vi "Parse Custom Mode (Pixhawk).vi"(8 "Error In":errorcluster, 11 "custom mode":u32) -> (0 "Error Out":errorcluster, 3 "Custom Mode":string)   [LabVIEW 2014]
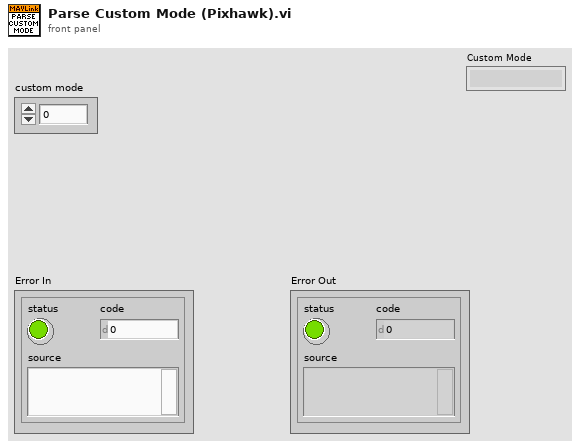
[diagram p1: front panel]
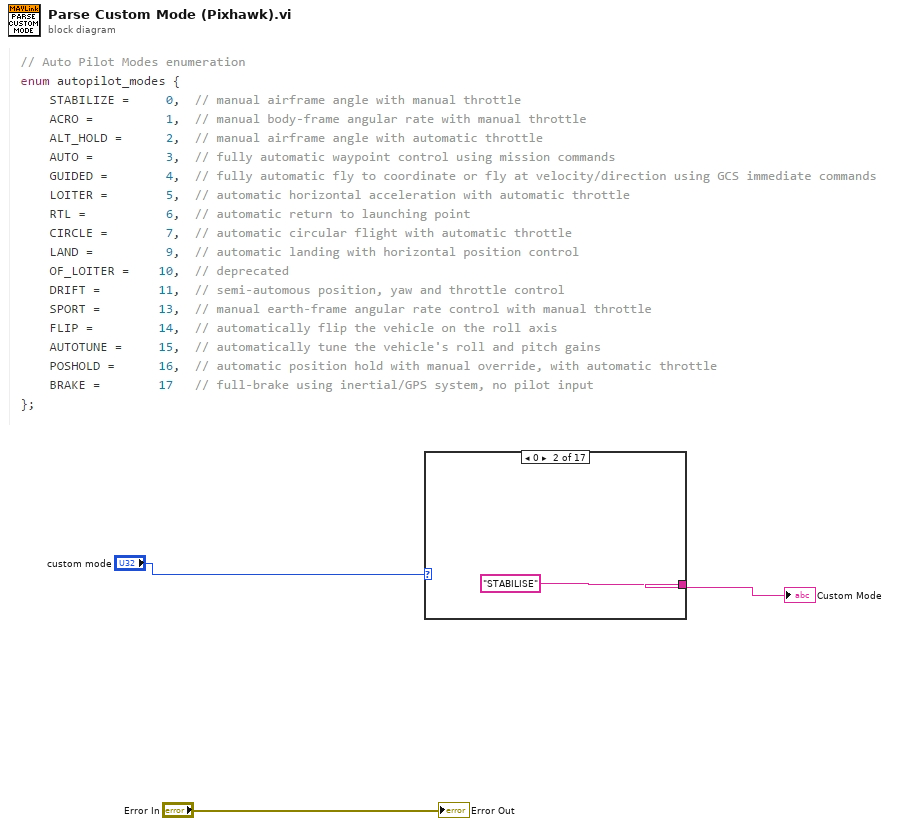
[diagram p0: block diagram]
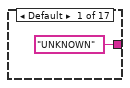
[diagram p2: hidden frame]
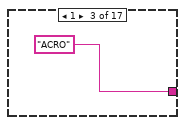
[diagram p3: hidden frame]
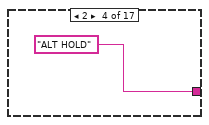
[diagram p4: hidden frame]
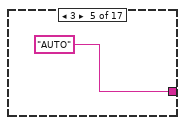
[diagram p5: hidden frame]
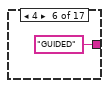
[diagram p6: hidden frame]
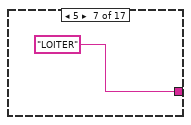
[diagram p7: hidden frame]
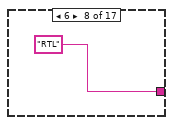
[diagram p8: hidden frame]
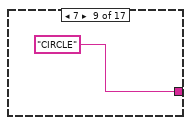
[diagram p9: hidden frame]
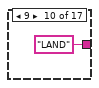
[diagram p10: hidden frame]
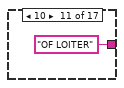
[diagram p11: hidden frame]
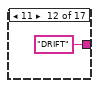
[diagram p12: hidden frame]
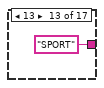
[diagram p13: hidden frame]
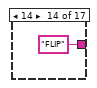
[diagram p14: hidden frame]
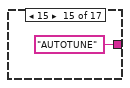
[diagram p15: hidden frame]
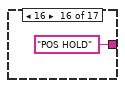
[diagram p16: hidden frame]
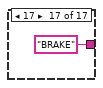
[diagram p17: hidden frame]
diagram:
  n1 = case shown="0" "custom mode" {
    tunnel: ["UNKNOWN" "STABILISE" "ACRO" "ALT HOLD" "AUTO" "GUIDED" "LOITER" "RTL" "CIRCLE" "LAND" "OF LOITER" "DRIFT" "SPORT" "FLIP" "AUTOTUNE" "POS HOLD" "BRAKE"] -> w2
    frame Default {
    }
    frame 0 {
    }
    frame 1 {
    }
    frame 2 {
    }
    frame 3 {
    }
    frame 4 {
    }
    frame 5 {
    }
    frame 6 {
    }
    frame 7 {
    }
    frame 9 {
    }
    frame 10 {
    }
    frame 11 {
    }
    frame 13 {
    }
    frame 14 {
    }
    frame 15 {
    }
    frame 16 {
    }
    frame 17 {
    }
  }
  "Custom Mode" <- w2
  "Error Out" <- "Error In"
